vi "test_generic.vi"() -> ()   [LabVIEW 2010, in "GenericImageProcessor.lvclass"]
uses:
  GenericImageProcessor.lvclass
  common/classes/Image/Image/Image.lvclass
  common/classes/GenericComponent/GenericComponent/GenericComponent.lvclass
panel:
  in  "createButton":bool
  in  "configure":bool
  in  "number of channels":i32=3
  in  "load image":bool
  out "image":T1[](array[plugin-control])
  in  "process":bool
  in  "stop":bool
  in  "adjust":bool
  # "Test console for ImageProcessors"
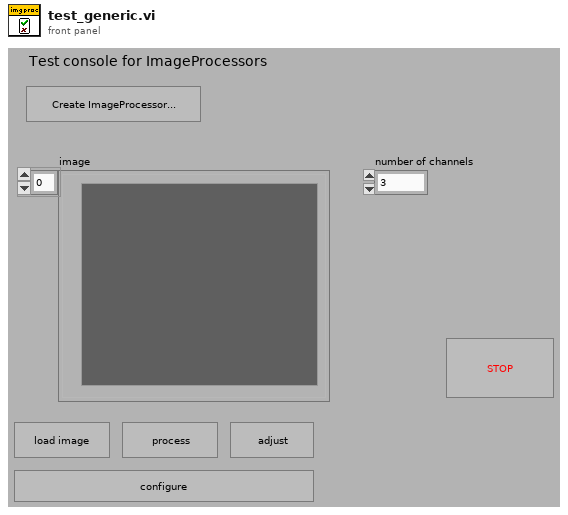
[diagram p1: front panel]
types:
  T1 = typedef "IMAQ Image.ctl" = refnum<image>
  T2 = typedef "XComponentSpecification.xctl/data.ctl" = cluster{"class path":string, "configuration":string, "label":string, "settings name":string}
  T3 = typedef "Image Type" = u32
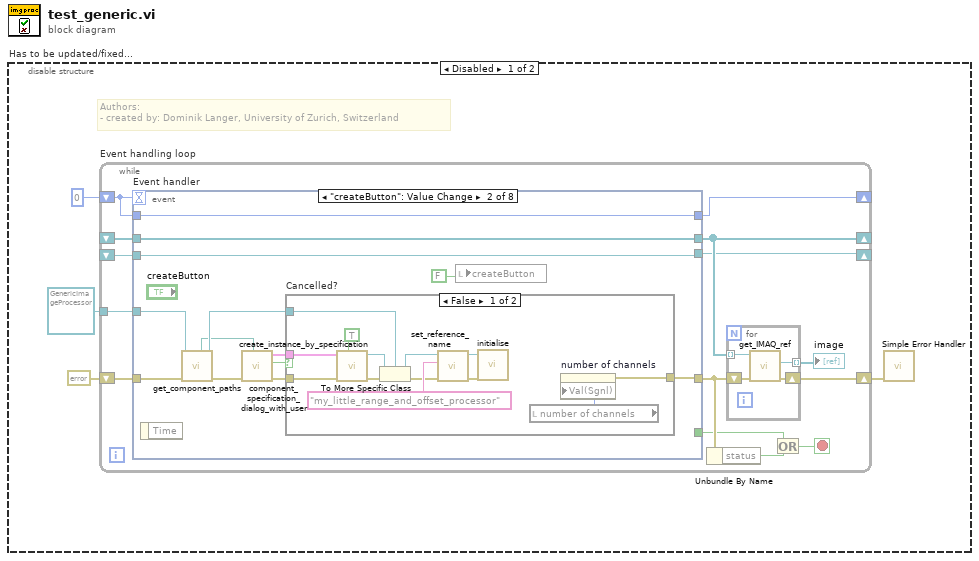
[diagram p0: block diagram]
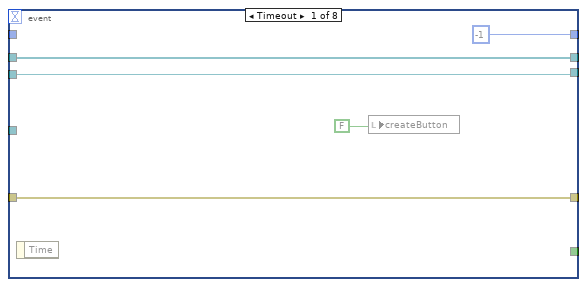
[diagram p2: hidden frame]
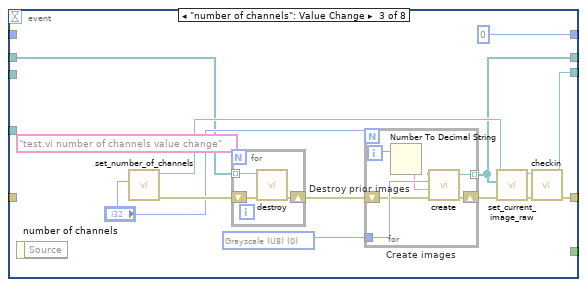
[diagram p4: hidden frame]
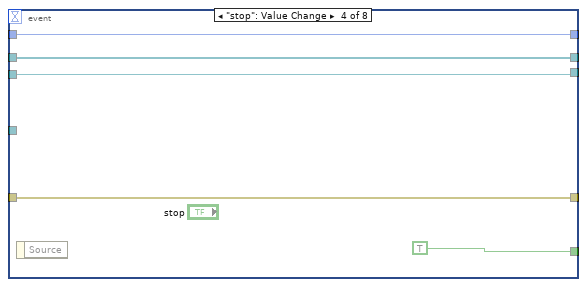
[diagram p5: hidden frame]
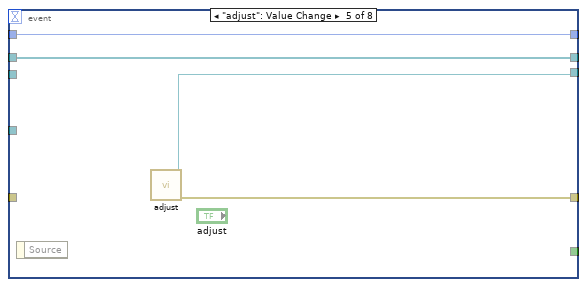
[diagram p6: hidden frame]
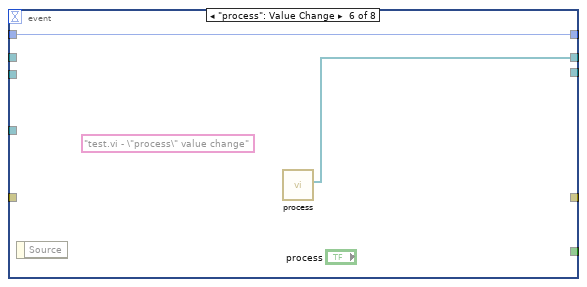
[diagram p7: hidden frame]
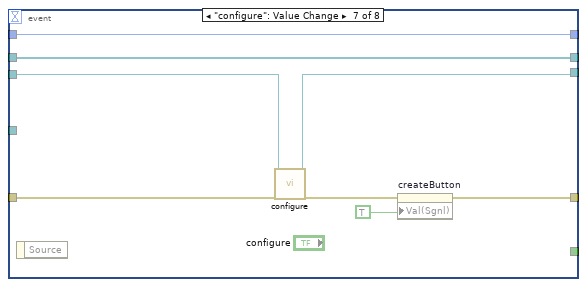
[diagram p8: hidden frame]
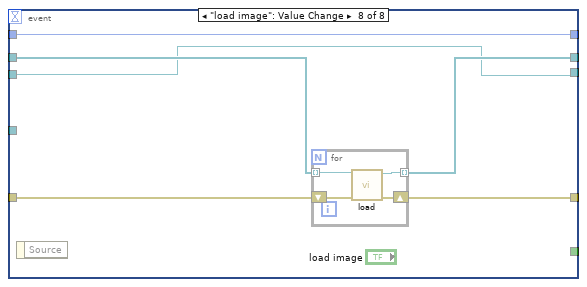
[diagram p9: hidden frame]
diagram:
  n1 = disable-structure "Has to be updated/fixed..." shown="Disabled" {
    frame Disabled {
      # "Authors: \n- created by: Dominik Langer, University of Zurich, Switzerland"
      n2 = while "Event handling loop" {
        shift-right: [w12] -> w3
        shift-left: errorcluster {"status"=FALSE, "code"=0, "source"=""} ("error out") -> [w18]
        shift-right: [w16] -> _
        shift-left: 0 -> [w17]
        shift-right: [w14] -> _
        shift-left: _ -> [w15]
        shift-right: [w6] -> _
        shift-left: _ -> [w7]
        tunnel: refnum<class "GenericImageProcessor.lvclass"> refnum ("GenericImageProcessor.lvclass") -> [w5]
        stop <- w8 stop-if-true
        n3 = event "Event handler" shown="[1] \"createButton\": Value Change" {
          selector: _ -> [_ _ _ _ _ _ _ _]
          dyn-events: _ -> [_ _ _ _ _ _ _ _]
          timeout: w17 -> [_ _ _ _ _ _ _ _]
          tunnel: w18 -> [w23 w32 w71 w86 w88 w101 w109 w116]
          tunnel: [-1 w40 0 w85 w92 w103 w111 w117] -> w16
          tunnel: w17 -> [_ w40 _ w85 w92 w103 w111 w117]
          tunnel: [_ _ _ TRUE _ _ _ _] -> w9
          tunnel: [w26 w39 w56 w83 w90 w102 w110 w114] -> w14
          tunnel: w15 -> [w26 w39 w57 w83 w90 _ w110 w115]
          tunnel: [w23 w37 w69 w86 w91 w96 w105 w113] -> w11
          tunnel: w7 -> [w25 w38 w67 w82 w87 w99 w108 w112]
          tunnel: [w25 w38 w65 w82 w89 w94 w107 w112] -> w6
          tunnel: w5 -> [_ w30 _ _ _ _ _ _]
          event Timeout {
            n4 = event-data() -> ()  [unwired: 2 out]
            n5 = local write "createButton"(FALSE) -> ()
          }
          event "createButton": Value Change {
            n6 = event-data() -> ()  [unwired: 2 out]
            n7 = call-dynamic "get_component_paths.vi"("error in (no error)"=w32, "GenericComponent in"=w30) -> ("error out"=w31:errorcluster, "GenericComponent out"=w29:refnum<class "GenericImageProcessor.lvclass">, "component type directory"=w28:path)  [unwired: 4 in, 3 out]
            n8 = call "component_specification_dialog_with_user.vi"("start path"=w28, "error in (no error)"=w31) -> ("error out"=w36:errorcluster, "cancelled?"=w33:bool, "component specification out"=w35:T2)  [unwired: 7 in]
            n9 = case "Cancelled?" shown="False" w33 {
              tunnel: w29 -> [w51 _]
              tunnel: [w44 w54] -> w37
              tunnel: w36 -> [w42 w54]
              tunnel: w35 -> [w41 _]
              frame False {
                n10 = call "create_instance_by_specification.vi"("call constructor?"=TRUE, "error in (no error)"=w42, "component specification"=w41) -> ("error out"=w52:errorcluster, "GenericPlugin out"=w53:refnum<class "GenericComponent.lvclass">)  [unwired: 6 in, 1 out]
                n11 = To More Specific Class(target class=w51, reference=w53, error in=w52) -> (specific class reference=w45:refnum<class "GenericImageProcessor.lvclass">, error out=w48:errorcluster)
                n12 = call "set_reference_name.vi"("error in (no error)"=w48, "reference name"="my_little_range_and_offset_processor", "GenericPlugin.lvclass in"=w45) -> ("error out"=w47:errorcluster, "GenericPlugin.lvclass out"=w46:refnum<class "GenericImageProcessor.lvclass">)  [unwired: 7 in]
                n13 = call-dynamic "initialise.vi"("error in (no error)"=w47, "GenericImageProcessor in"=w46) -> ()  [unwired: 10 out]
                n14 = local read "number of channels"() -> (w43:i32)
                n15 = property on="number of channels" class="DigNum (strict)"("Val(Sgnl)"=w43) -> (error out=w44:errorcluster)  [unwired: 2 in, 1 out]
              }
              frame True {
              }
            }
            n16 = local write "createButton"(FALSE) -> ()
          }
          event "number of channels": Value Change {
            w64 = T3 0 items=["Grayscale (U8)", "Grayscale (I16)", "Grayscale (SGL)", "Complex (CSG)", "RGB (U32)", "HSL (U32)", "RGB (U64)", "Grayscale (U16)"] ("Image Type")
            w68 = "test.vi number of channels value change" ("locked by?")
            n17 = event-data() -> ()  [unwired: 2 out]
            n18 = call "set_number_of_channels.vi"("number of channels"="number of channels") -> ("error out"=w60:errorcluster, "GenericImageProcessor.lvclass out"=w58:refnum<class "GenericImageProcessor.lvclass">, "error in (no error)"=w70:errorcluster, "GenericImageProcessor.lvclass in"=w66:refnum<class "GenericImageProcessor.lvclass">)  [unwired: 7 out]
            n19 = for "Destroy prior images" {
              shift-right: [w74] -> w63
              shift-left: w60 -> [w75]
              tunnel: w57 -> [w73] mode=indexing
              n20 = call-dynamic "destroy.vi"("error in (no error)"=w75, "Image in"=w73) -> ("error out"=w74:errorcluster)  [unwired: 9 out]
            }
            n21 = for "Create images" {
              N: "number of channels" -> [_]
              tunnel: [w78] -> w56 mode=indexing
              shift-right: [w79] -> w62
              shift-left: w63 -> [w80]
              tunnel: w64 -> [w81]
              i -> [w77]
              n22 = Number To Decimal String(number=w77) -> (decimal integer string=w76:string)  [unwired: 1 out]
              n23 = call "create.vi"("error in (no error)"=w80, "name"=w76, "Image Type"=w81) -> ("error out"=w79:errorcluster, "Image out"=w78:refnum<class "Image.lvclass">)  [unwired: 1 in, 6 out]
            }
            n24 = call-dynamic "set_current_image_raw.vi"("error in (no error)"=w62, "current image raw (channels)"=w56, "GenericImageProcessor.lvclass in"=w58) -> ("error out"=w61:errorcluster, "GenericImageProcessor.lvclass out"=w55:refnum<class "GenericImageProcessor.lvclass">)  [unwired: 7 out]
            n25 = call-dynamic "checkin.vi"("error in (no error)"=w61, "GenericImageProcessor in"=w55) -> ("error out"=w69:errorcluster, "GenericImageProcessor out"=w65:refnum<class "GenericImageProcessor.lvclass">)  [unwired: 8 out]
          }
          event "stop": Value Change {
            n26 = event-data() -> ()  [unwired: 2 out]
          }
          event "adjust": Value Change {
            n27 = event-data() -> ()  [unwired: 2 out]
            n28 = call-dynamic "adjust.vi"() -> ("error out"=w91:errorcluster, "GenericImageProcessor out"=w89:refnum<class "GenericImageProcessor.lvclass">)  [unwired: 2 in, 8 out]
          }
          event "process": Value Change {
            w93 = "test.vi - \"process\" value change" ("locked by?")
            n29 = event-data() -> ()  [unwired: 2 out]
            n30 = call-dynamic "process.vi"() -> ("error out"=w97:errorcluster, "destination image out (channels)"=w102:refnum<class "Image.lvclass">[], "GenericImageProcessor out"=w95:refnum<class "GenericImageProcessor.lvclass">, "error in (no error)"=w100:errorcluster, "GenericImageProcessor in"=w98:refnum<class "GenericImageProcessor.lvclass">)  [unwired: 1 in, 6 out]
          }
          event "configure": Value Change {
            n31 = event-data() -> ()  [unwired: 2 out]
            n32 = call-dynamic "configure.vi"("error in (no error)"=w109, "GenericPlugin in"=w108) -> ("error out"=w106:errorcluster, "GenericPlugin out"=w107:refnum<class "GenericImageProcessor.lvclass">)  [unwired: 8 out]
            n33 = property on="createButton" class="Bool (strict)"(error in=w106, "Val(Sgnl)"=TRUE) -> (error out=w105:errorcluster)  [unwired: 1 in, 1 out]
          }
          event "load image": Value Change {
            n34 = event-data() -> ()  [unwired: 2 out]
            n35 = for {
              tunnel: w115 -> [w120] mode=indexing
              tunnel: [w119] -> w114 mode=indexing
              shift-right: [w118] -> w113
              shift-left: w116 -> [w121]
              n36 = call-dynamic "load.vi"("error in (no error)"=w121, "Image in"=w120) -> ("error out"=w118:errorcluster, "Image out"=w119:refnum<class "Image.lvclass">)  [unwired: 2 in, 6 out]
            }
          }
        }
        n37 = Unbundle By Name(w11) -> ("status"=w10:bool)
        n38 = for {
          tunnel: w14 -> [w21] mode=indexing
          shift-right: [w20] -> w12
          shift-left: w11 -> [w22]
          tunnel: [w19] -> w13 mode=indexing
          n39 = call-dynamic "get_IMAQ_ref.vi"("error in (no error)"=w22, "Image.lvclass in"=w21) -> ("error out"=w20:errorcluster, "Image"=w19:T1)  [unwired: 8 out]
        }
        "image" <- w13
        n40 = Or(x=w9, y=w10) -> (x .or. y?=w8:bool)
      }
      n41 = call <vilib>:"Simple Error Handler.vi"("error in (no error)"=w3) -> ()  [unwired: 1 in, 8 out]
    }
    frame Enabled {
    }
  }
